vi "AES Encrypt (CBC).vi"(7 "Padding":i32(ring)=3 items=["None"=1, "PKCS7"=2, "Zeros"=3, "ANSIX923"=4, "ISO10126"=5], 8 "error in (no error)":errorcluster, 9 "IV":u8[](array[numeric]), 10 "Key":u8[](array[numeric]), 11 "Raw data in":u8[](array[numeric])) -> (0 "error out":errorcluster, 1 "IV out":u8[](array[numeric]), 3 "Encrypted data out":u8[](array[numeric]))   [LabVIEW 2021, in "dotNET Crypto Symmetric Encryption.lvlib"]
doc: "Encrypt data using AES using the CBC cipher mode. \n\nA suitable padding mode should be used if the data length does not match a multiple of the block size. The same padding mode must be selected when decrypting the data.\n\nThe IV (Initialisation Vector) can be left blank to be automatically generated. The IV must be available/stored for decryption of the data."
uses:
  dotNET Crypto Symmetric Encryption.lvlib
  System.Core
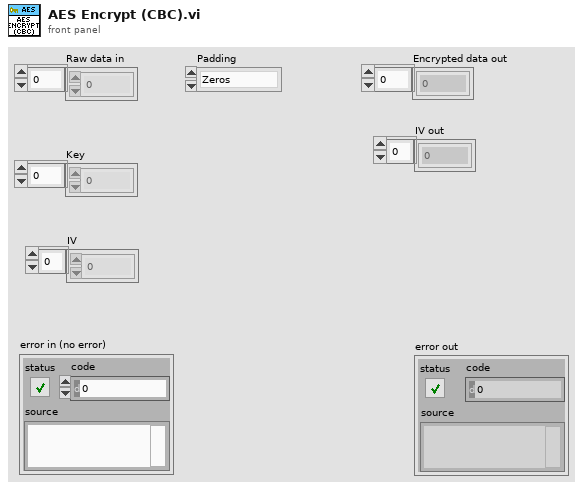
[diagram p1: front panel]
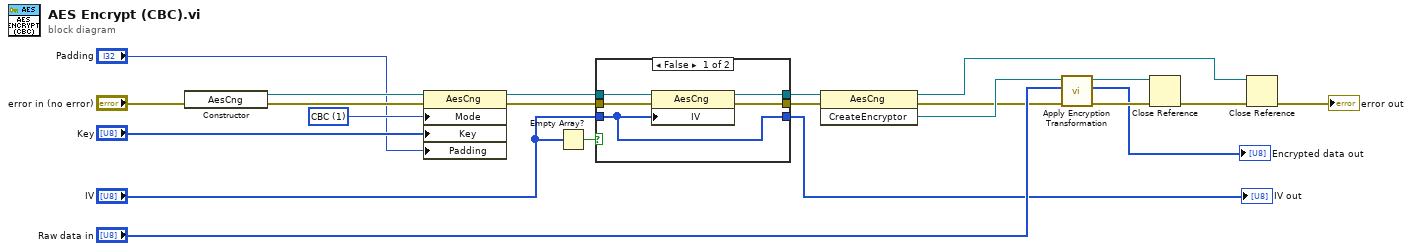
[diagram p0: block diagram]
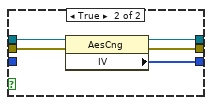
[diagram p2: hidden frame]
diagram:
  w20 = 1 items=["CBC"=1, "ECB"=2, "OFB"=3, "CFB"=4, "CTS"=5] ("Mode")
  n1 = constructor class="AesCng"(error in="error in (no error)") -> (reference out=w17:refnum<k24>, error out=w18:errorcluster)  [unwired: 2 in, 1 out]
  n2 = property class="AesCng"(reference=w17, error in=w18, "Mode"=w20, "Key"="Key", "Padding"="Padding") -> (reference out=w7:refnum<k24>, error out=w5:errorcluster)
  n3 = Empty Array?(array="IV") -> (empty?=w3:bool)
  n4 = case shown="False" w3 {
    tunnel: w7 -> [w27 w32]
    tunnel: [w26 w29] -> w6
    tunnel: w5 -> [w25 w31]
    tunnel: [w24 w30] -> w4
    tunnel: "IV" -> [w23 _]
    tunnel: [w23 w28] -> w1
    frame False {
      n5 = property class="AesCng"(reference=w27, error in=w25, "IV"=w23) -> (reference out=w26:refnum<k24>, error out=w24:errorcluster)
    }
    frame True {
      n6 = property class="AesCng"(reference=w32, error in=w31) -> (reference out=w29:refnum<k24>, error out=w30:errorcluster, "IV"=w28:u8[])
    }
  }
  "IV out" <- w1
  n7 = invoke class="AesCng" method="CreateEncryptor"(reference=w6, error in=w4) -> (reference out=w13:refnum<k24>, error out=w12:errorcluster, "CreateEncryptor"=w19:refnum<k24>)  [unwired: 1 in]
  n8 = call "Apply Encryption Transformation.vi"("error in (no error)"=w12, "Raw data in"="Raw data in", "CryptoTransform in"=w19) -> ("error out"=w15:errorcluster, "Encrypted data out"=→"Encrypted data out":u8[], "CryptoTransform out"=w10:refnum<k24>)  [unwired: 6 in]
  n9 = Close Reference(reference=w10, error in (no error)=w15) -> (error out=w11:errorcluster)
  n10 = Close Reference(reference=w13, error in (no error)=w11) -> (error out=→"error out":errorcluster)
